vi "Tosca-Setup Session Metadata.vi"(0 "Session Info":T3, 7 "Path":path=path "C:/Data/Tosca/ToscaMetadata.cs") -> (4 "Metadata":string, 8 "Canceled?":bool)   [LabVIEW 2020]
uses:
  epl-vi-lib/Utility VIs/Controls/KPropertyTable/KPropertyTable.xctl
panel:
  in  "Tab":enum32{"CS", "M"}(tab)
  in  "Table":T1[](xcontrol)
  out "Session String":string
  out "exit signal":bool
  in  "Cancel":bool
  in  "OK":bool
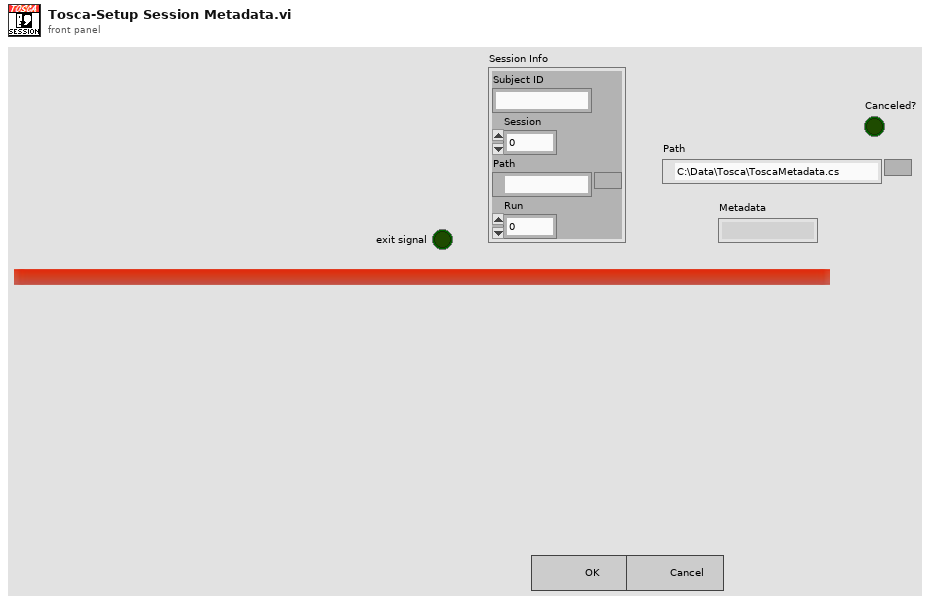
[diagram p1: front panel]
types:
  T1 = typedef "KPropertyTable.xctl/RowData.ctl" = cluster{"Name":string, "Type":T2, "Category":string, "Strings":string[], "Value":string}
  T2 = typedef "KPropertyTable.xctl/DataType.ctl" = enum16{"String", "Enum", "Int", "Double", "Boolean", "Ring", "Formula"}
  T3 = cluster{"Subject ID":string, "Session":i32, "Path":path, "Run":i32}
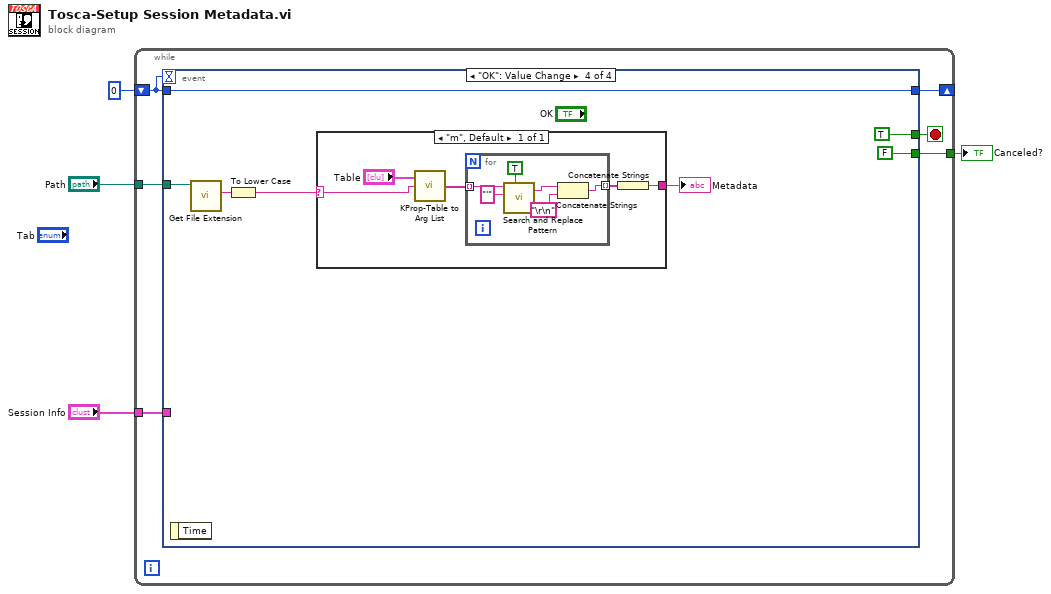
[diagram p0: block diagram]
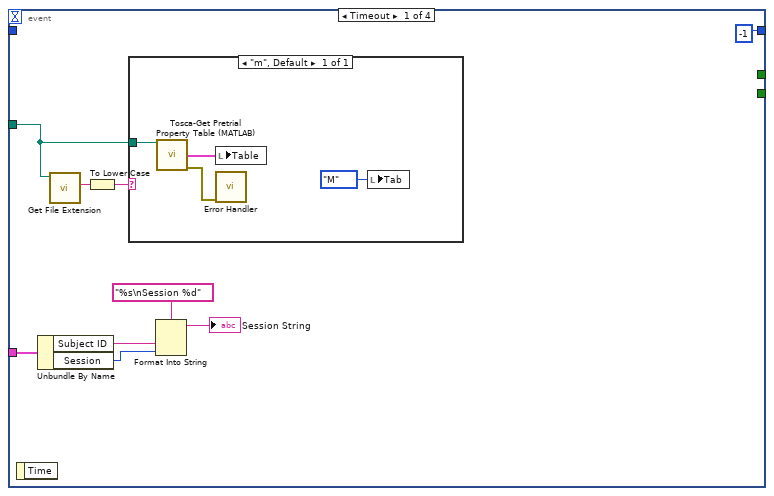
[diagram p2: hidden frame]
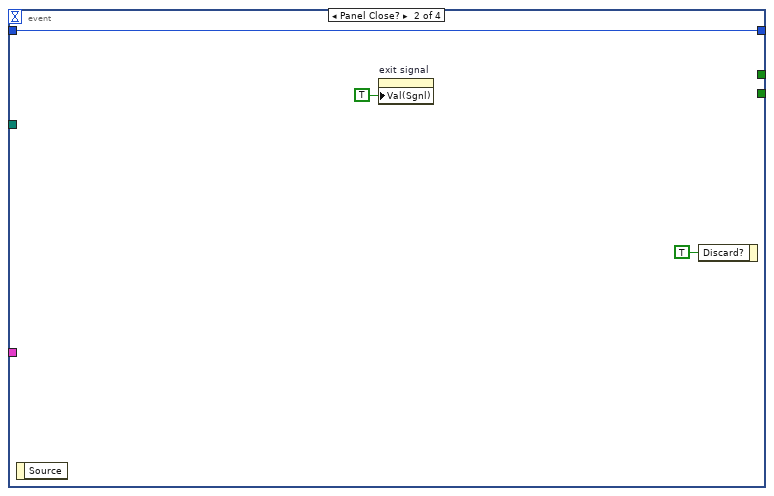
[diagram p3: hidden frame]
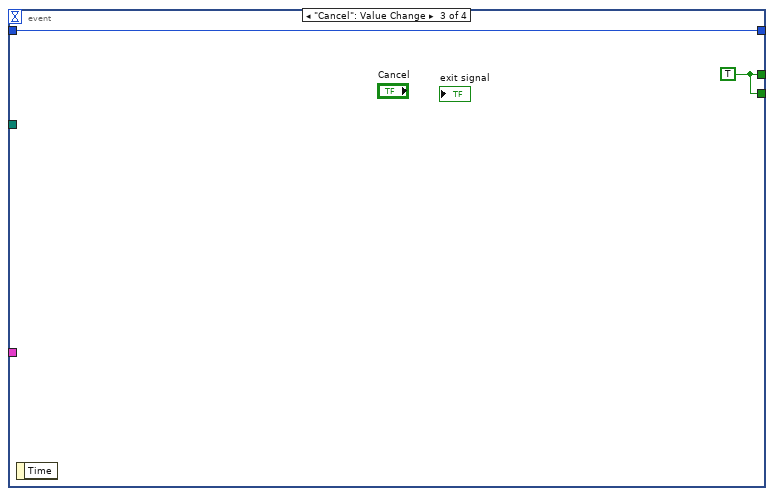
[diagram p4: hidden frame]
diagram:
  n1 = while {
    shift-right: [w10] -> _
    shift-left: 0 -> [w7]
    tunnel: [w8] -> w3
    tunnel: "Path" -> [w6]
    tunnel: "Session Info" -> [w5]
    stop <- w9 stop-if-true
    n2 = event shown="[3] \"OK\": Value Change" {
      selector: _ -> [_ _ _ _]
      dyn-events: _ -> [_ _ _ _]
      timeout: w7 -> [_ _ _ _]
      tunnel: [-1 w26 w27 w33] -> w10
      tunnel: [_ _ w28 TRUE] -> w9
      tunnel: [_ _ w28 FALSE] -> w8
      tunnel: w7 -> [_ w26 w27 w33]
      tunnel: w6 -> [w13 _ _ w30]
      tunnel: w5 -> [w18 _ _ _]
      event Timeout {
        n3 = event-data() -> ()  [unwired: 1 in, 1 out]
        n4 = Unbundle By Name(w18) -> ("Subject ID"=w16:string, "Session"=w15:i32)
        n5 = call <vilib>:"Get File Extension.vi"("file"=w13) -> ("lowercase file extension"=w12:string)  [unwired: 6 in, 4 out]
        n6 = To Lower Case(string=w12) -> (all lower case string=w11:string)
        n7 = case shown="\"m\", Default" w11 {
          tunnel: w13 -> [w22]
          frame "m", Default {
            n8 = call "Tosca-Get Pretrial Property Table (MATLAB).vi"("Path"=w22) -> ("Table"=w21:T1[], "error out"=w20:errorcluster)  [unwired: 13 in]
            n9 = local write "Table"(w21) -> ()
            n10 = call "Error Handler.vi"("error in (no error)"=w20) -> ()  [unwired: 13 in, 2 out]
            n11 = local write "Tab"(enum32{"CS", "M"}."M" ("Tab")) -> ()
          }
        }
        n12 = Format Into String(format string="%s\nSession %d", w16, w15) -> (resulting string=→"Session String":string)  [unwired: 2 in, 1 out]
      }
      event Panel Close? {
        n13 = event-data() -> ()  [unwired: 1 in, 1 out]
        n14 = property on="exit signal" class="Bool (strict)"("Val(Sgnl)"=TRUE ("Value (Signaling)")) -> ()  [unwired: 2 in, 2 out]
        n15 = event-data("Discard?"=TRUE) -> ()  [unwired: 1 in, 1 out]
      }
      event "Cancel": Value Change {
        w28 = TRUE
        n16 = event-data() -> ()  [unwired: 1 in, 1 out]
      }
      event "OK": Value Change {
        n17 = event-data() -> ()  [unwired: 1 in, 1 out]
        n18 = call <vilib>:"Get File Extension.vi"("file"=w30) -> ("lowercase file extension"=w31:string)  [unwired: 6 in, 4 out]
        n19 = To Lower Case(string=w31) -> (all lower case string=w29:string)
        n20 = case shown="\"m\", Default" w29 {
          selector: w29 -> [w39]
          tunnel: [w36] -> w32
          frame "m", Default {
            n21 = call "KProp-Table to Arg List.vi"("Rows"="Table", "type"=w39) -> ("Args"=w38:string[])  [unwired: 13 in]
            n22 = for {
              tunnel: w38 -> [w44] mode=indexing
              tunnel: [w45] -> w37 mode=indexing
              n23 = call <vilib>:"Search and Replace Pattern.vi"("string"=w44, "regular expression (\"\")"="'" ("regular expression (\"\")"), "replace all? (F)"=TRUE) -> ("result string"=w43:string)  [unwired: 2 in, 1 out]
              n24 = Concatenate Strings(w43, "\r\n") -> (w45:string)
            }
            n25 = Concatenate Strings(w37) -> (w36:string)
          }
        }
        "Metadata" <- w32
      }
    }
  }
  "Canceled?" <- w3
